vi "SIAM-7xRollingShutter.vi"() -> ()   [LabVIEW 2011]
uses:
  SIAM_command.ctl
panel:
  in  "Wob/µm":dbl=63.28
  in  "Grid µm":dbl=29.0
  out "set Camera Exposure [µs]":dbl=743.175
  in  "PhaseImages":u16=7
  in  "GalvoX-Blanking":dbl
  in  "NoOfImages":u16=35
  out "µmShift":dbl=10.96096971726759 format="%#_8g"
  in  "Camera-Lines":u32=1082
  in  "Turn_ticks":u32=120
  in  "SM_ticks":u32=116
  in  "Trigger_ticks":u32=100
  in  "Mask_tpos":dbl=45853.0
  in  "LineTime-µs":dbl=27.525
  in  "RollingShutter height":u16=27
  in  "galvox/pixel":dbl=7.407
  in  "galvox-Line1080":dbl=-12220.0
  out "SIAMScript":T2(array[cluster])=[{"Delay 10µs"=50, "command"=1612709953, "P0"=0, "P1"=-269103235, "P2"=0, "P3"=0, "P4"=0, "P5-ticket"=0}, {"Delay 10µs"=0, "command"=1611661377, "P0"=0, "P1"=0, "P2"=0, "P3"=0, "P4"=0, "P5-ticket"=0}, {"Delay 10µs"=120, "command"=1612709921, "P0"=0, "P1"=0, "P2"=-2821727, "P3"=0, "P4"=0, "P5-ticket"=0}, {"Delay 10µs"=113, "command"=3506438145, "P0"=1, "P1"=1, "P2"=0, "P3"=0, "P4"=0, "P5-ticket"=0}, {"Delay 10µs"=100, "command"=3506438145, "P0"=1, "P1"=0, "P2"=0, "P3"=0, "P4"=0, "P5-ticket"=0}, {"Delay 10µs"=2856, "command"=1612709921, "P0"=0, "P1"=0, "P2"=0, "P3"=0, "P4"=0, "P5-ticket"=0}, {"Delay 10µs"=50, "command"=1612709953, "P0"=0, "P1"=-269103235, "P2"=0, "P3"=0, "P4"=0, "P5-ticket"=0}, {"Delay 10µs"=0, "command"=1611661377, "P0"=0, "P1"=45250435, "P2"=0, "P3"=0, "P4"=0, "P5-ticket"=0}, {"Delay 10µs"=120, "command"=1612709921, "P0"=0, "P1"=0, "P2"=-2821727, "P3"=0, "P4"=0, "P5-ticket"=0}, {"Delay 10µs"=113, "command"=3506438145, "P0"=1, "P1"=1, "P2"=0, "P3"=0, "P4"=0, "P5-ticket"=0}, {"Delay 10µs"=100, "command"=3506438145, "P0"=1, "P1"=0, "P2"=0, "P3"=0, "P4"=0, "P5-ticket"=0}, {"Delay 10µs"=2856, "command"=1612709921, "P0"=0, "P1"=0, "P2"=0, "P3"=0, "P4"=0, "P5-ticket"=0}, {"Delay 10µs"=50, "command"=1612709953, "P0"=0, "P1"=-269103235, "P2"=0, "P3"=0, "P4"=0, "P5-ticket"=0}, {"Delay 10µs"=0, "command"=1611661377, "P0"=0, "P1"=90500870, "P2"=0, "P3"=0, "P4"=0, "P5-ticket"=0}, {"Delay 10µs"=120, "command"=1612709921, "P0"=0, "P1"=0, "P2"=-2821727, "P3"=0, "P4"=0, "P5-ticket"=0}, {"Delay 10µs"=113, "command"=3506438145, "P0"=1, "P1"=1, "P2"=0, "P3"=0, "P4"=0, "P5-ticket"=0}, {"Delay 10µs"=100, "command"=3506438145, "P0"=1, "P1"=0, "P2"=0, "P3"=0, "P4"=0, "P5-ticket"=0}, {"Delay 10µs"=2856, "command"=1612709921, "P0"=0, "P1"=0, "P2"=0, "P3"=0, "P4"=0, "P5-ticket"=0}, {"Delay 10µs"=50, "command"=1612709953, "P0"=0, "P1"=-269103235, "P2"=0, "P3"=0, "P4"=0, "P5-ticket"=0}, {"Delay 10µs"=0, "command"=1611661377, "P0"=0, "P1"=135751305, "P2"=0, "P3"=0, "P4"=0, "P5-ticket"=0}, {"Delay 10µs"=120, "command"=1612709921, "P0"=0, "P1"=0, "P2"=-2821727, "P3"=0, "P4"=0, "P5-ticket"=0}, {"Delay 10µs"=113, "command"=3506438145, "P0"=1, "P1"=1, "P2"=0, "P3"=0, "P4"=0, "P5-ticket"=0}, {"Delay 10µs"=100, "command"=3506438145, "P0"=1, "P1"=0, "P2"=0, "P3"=0, "P4"=0, "P5-ticket"=0}, {"Delay 10µs"=2856, "command"=1612709921, "P0"=0, "P1"=0, "P2"=0, "P3"=0, "P4"=0, "P5-ticket"=0}, {"Delay 10µs"=50, "command"=1612709953, "P0"=0, "P1"=-269103235, "P2"=0, "P3"=0, "P4"=0, "P5-ticket"=0}, {"Delay 10µs"=0, "command"=1611661377, "P0"=0, "P1"=181001740, "P2"=0, "P3"=0, "P4"=0, "P5-ticket"=0}, {"Delay 10µs"=120, "command"=1612709921, "P0"=0, "P1"=0, "P2"=-2821727, "P3"=0, "P4"=0, "P5-ticket"=0}, {"Delay 10µs"=113, "command"=3506438145, "P0"=1, "P1"=1, "P2"=0, "P3"=0, "P4"=0, "P5-ticket"=0}, {"Delay 10µs"=100, "command"=3506438145, "P0"=1, "P1"=0, "P2"=0, "P3"=0, "P4"=0, "P5-ticket"=0}, {"Delay 10µs"=2856, "command"=1612709921, "P0"=0, "P1"=0, "P2"=0, "P3"=0, "P4"=0, "P5-ticket"=0}, {"Delay 10µs"=50, "command"=1612709953, "P0"=0, "P1"=-269103235, "P2"=0, "P3"=0, "P4"=0, "P5-ticket"=0}, {"Delay 10µs"=0, "command"=1611661377, "P0"=0, "P1"=226252175, "P2"=0, "P3"=0, "P4"=0, "P5-ticket"=0}, {"Delay 10µs"=120, "command"=1612709921, "P0"=0, "P1"=0, "P2"=-2821727, "P3"=0, "P4"=0, "P5-ticket"=0}, {"Delay 10µs"=113, "command"=3506438145, "P0"=1, "P1"=1, "P2"=0, "P3"=0, "P4"=0, "P5-ticket"=0}, {"Delay 10µs"=100, "command"=3506438145, "P0"=1, "P1"=0, "P2"=0, "P3"=0, "P4"=0, "P5-ticket"=0}, {"Delay 10µs"=2856, "command"=1612709921, "P0"=0, "P1"=0, "P2"=0, "P3"=0, "P4"=0, "P5-ticket"=0}, {"Delay 10µs"=50, "command"=1612709953, "P0"=0, "P1"=-269103235, "P2"=0, "P3"=0, "P4"=0, "P5-ticket"=0}, {"Delay 10µs"=0, "command"=1611661377, "P0"=0, "P1"=271502610, "P2"=0, "P3"=0, "P4"=0, "P5-ticket"=0}, {"Delay 10µs"=120, "command"=1612709921, "P0"=0, "P1"=0, "P2"=-2821727, "P3"=0, "P4"=0, "P5-ticket"=0}, {"Delay 10µs"=113, "command"=3506438145, "P0"=1, "P1"=1, "P2"=0, "P3"=0, "P4"=0, "P5-ticket"=0}, {"Delay 10µs"=100, "command"=3506438145, "P0"=1, "P1"=0, "P2"=0, "P3"=0, "P4"=0, "P5-ticket"=0}, {"Delay 10µs"=2856, "command"=1612709921, "P0"=0, "P1"=0, "P2"=0, "P3"=0, "P4"=0, "P5-ticket"=0}, {"Delay 10µs"=50, "command"=1612709953, "P0"=0, "P1"=-269103235, "P2"=0, "P3"=0, "P4"=0, "P5-ticket"=0}, {"Delay 10µs"=0, "command"=1611661377, "P0"=0, "P1"=316753045, "P2"=0, "P3"=0, "P4"=0, "P5-ticket"=0}, {"Delay 10µs"=120, "command"=1612709921, "P0"=0, "P1"=0, "P2"=-2821727, "P3"=0, "P4"=0, "P5-ticket"=0}, {"Delay 10µs"=113, "command"=3506438145, "P0"=1, "P1"=1, "P2"=0, "P3"=0, "P4"=0, "P5-ticket"=0}, {"Delay 10µs"=100, "command"=3506438145, "P0"=1, "P1"=0, "P2"=0, "P3"=0, "P4"=0, "P5-ticket"=0}, {"Delay 10µs"=2856, "command"=1612709921, "P0"=0, "P1"=0, "P2"=0, "P3"=0, "P4"=0, "P5-ticket"=0}, {"Delay 10µs"=50, "command"=1612709953, "P0"=0, "P1"=-269103235, "P2"=0, "P3"=0, "P4"=0, "P5-ticket"=0}, {"Delay 10µs"=0, "command"=1611661377, "P0"=0, "P1"=362003480, "P2"=0, "P3"=0, "P4"=0, "P5-ticket"=0}, {"Delay 10µs"=120, "command"=1612709921, "P0"=0, "P1"=0, "P2"=-2821727, "P3"=0, "P4"=0, "P5-ticket"=0}, {"Delay 10µs"=113, "command"=3506438145, "P0"=1, "P1"=1, "P2"=0, "P3"=0, "P4"=0, "P5-ticket"=0}, {"Delay 10µs"=100, "command"=3506438145, "P0"=1, "P1"=0, "P2"=0, "P3"=0, "P4"=0, "P5-ticket"=0}, {"Delay 10µs"=2856, "command"=1612709921, "P0"=0, "P1"=0, "P2"=0, "P3"=0, "P4"=0, "P5-ticket"=0}, {"Delay 10µs"=50, "command"=1612709953, "P0"=0, "P1"=-269103235, "P2"=0, "P3"=0, "P4"=0, "P5-ticket"=0}, {"Delay 10µs"=0, "command"=1611661377, "P0"=0, "P1"=407253915, "P2"=0, "P3"=0, "P4"=0, "P5-ticket"=0}, {"Delay 10µs"=120, "command"=1612709921, "P0"=0, "P1"=0, "P2"=-2821727, "P3"=0, "P4"=0, "P5-ticket"=0}, {"Delay 10µs"=113, "command"=3506438145, "P0"=1, "P1"=1, "P2"=0, "P3"=0, "P4"=0, "P5-ticket"=0}, {"Delay 10µs"=100, "command"=3506438145, "P0"=1, "P1"=0, "P2"=0, "P3"=0, "P4"=0, "P5-ticket"=0}, {"Delay 10µs"=2856, "command"=1612709921, "P0"=0, "P1"=0, "P2"=0, "P3"=0, "P4"=0, "P5-ticket"=0}, {"Delay 10µs"=50, "command"=1612709953, "P0"=0, "P1"=-269103235, "P2"=0, "P3"=0, "P4"=0, "P5-ticket"=0}, {"Delay 10µs"=0, "command"=1611661377, "P0"=0, "P1"=452504350, "P2"=0, "P3"=0, "P4"=0, "P5-ticket"=0}, {"Delay 10µs"=120, "command"=1612709921, "P0"=0, "P1"=0, "P2"=-2821727, "P3"=0, "P4"=0, "P5-ticket"=0}, {"Delay 10µs"=113, "command"=3506438145, "P0"=1, "P1"=1, "P2"=0, "P3"=0, "P4"=0, "P5-ticket"=0}, {"Delay 10µs"=100, "command"=3506438145, "P0"=1, "P1"=0, "P2"=0, "P3"=0, "P4"=0, "P5-ticket"=0}, {"Delay 10µs"=2856, "command"=1612709921, "P0"=0, "P1"=0, "P2"=0, "P3"=0, "P4"=0, "P5-ticket"=0}, {"Delay 10µs"=50, "command"=1612709953, "P0"=0, "P1"=-269103235, "P2"=0, "P3"=0, "P4"=0, "P5-ticket"=0}, {"Delay 10µs"=0, "command"=1611661377, "P0"=0, "P1"=497754785, "P2"=0, "P3"=0, "P4"=0, "P5-ticket"=0}, {"Delay 10µs"=120, "command"=1612709921, "P0"=0, "P1"=0, "P2"=-2821727, "P3"=0, "P4"=0, "P5-ticket"=0}, {"Delay 10µs"=113, "command"=3506438145, "P0"=1, "P1"=1, "P2"=0, "P3"=0, "P4"=0, "P5-ticket"=0}, {"Delay 10µs"=100, "command"=3506438145, "P0"=1, "P1"=0, "P2"=0, "P3"=0, "P4"=0, "P5-ticket"=0}, {"Delay 10µs"=2856, "command"=1612709921, "P0"=0, "P1"=0, "P2"=0, "P3"=0, "P4"=0, "P5-ticket"=0}, {"Delay 10µs"=50, "command"=1612709953, "P0"=0, "P1"=-269103235, "P2"=0, "P3"=0, "P4"=0, "P5-ticket"=0}, {"Delay 10µs"=0, "command"=1611661377, "P0"=0, "P1"=543005220, "P2"=0, "P3"=0, "P4"=0, "P5-ticket"=0}, {"Delay 10µs"=120, "command"=1612709921, "P0"=0, "P1"=0, "P2"=-2821727, "P3"=0, "P4"=0, "P5-ticket"=0}, {"Delay 10µs"=113, "command"=3506438145, "P0"=1, "P1"=1, "P2"=0, "P3"=0, "P4"=0, "P5-ticket"=0}, {"Delay 10µs"=100, "command"=3506438145, "P0"=1, "P1"=0, "P2"=0, "P3"=0, "P4"=0, "P5-ticket"=0}, {"Delay 10µs"=2856, "command"=1612709921, "P0"=0, "P1"=0, "P2"=0, "P3"=0, "P4"=0, "P5-ticket"=0}, {"Delay 10µs"=50, "command"=1612709953, "P0"=0, "P1"=-269103235, "P2"=0, "P3"=0, "P4"=0, "P5-ticket"=0}, {"Delay 10µs"=0, "command"=1611661377, "P0"=0, "P1"=588255655, "P2"=0, "P3"=0, "P4"=0, "P5-ticket"=0}, {"Delay 10µs"=120, "command"=1612709921, "P0"=0, "P1"=0, "P2"=-2821727, "P3"=0, "P4"=0, "P5-ticket"=0}, {"Delay 10µs"=113, "command"=3506438145, "P0"=1, "P1"=1, "P2"=0, "P3"=0, "P4"=0, "P5-ticket"=0}, {"Delay 10µs"=100, "command"=3506438145, "P0"=1, "P1"=0, "P2"=0, "P3"=0, "P4"=0, "P5-ticket"=0}, {"Delay 10µs"=2856, "command"=1612709921, "P0"=0, "P1"=0, "P2"=0, "P3"=0, "P4"=0, "P5-ticket"=0}, {"Delay 10µs"=50, "command"=1612709953, "P0"=0, "P1"=-269103235, "P2"=0, "P3"=0, "P4"=0, "P5-ticket"=0}, {"Delay 10µs"=0, "command"=1611661377, "P0"=0, "P1"=633506090, "P2"=0, "P3"=0, "P4"=0, "P5-ticket"=0}, {"Delay 10µs"=120, "command"=1612709921, "P0"=0, "P1"=0, "P2"=-2821727, "P3"=0, "P4"=0, "P5-ticket"=0}, {"Delay 10µs"=113, "command"=3506438145, "P0"=1, "P1"=1, "P2"=0, "P3"=0, "P4"=0, "P5-ticket"=0}, {"Delay 10µs"=100, "command"=3506438145, "P0"=1, "P1"=0, "P2"=0, "P3"=0, "P4"=0, "P5-ticket"=0}, {"Delay 10µs"=2856, "command"=1612709921, "P0"=0, "P1"=0, "P2"=0, "P3"=0, "P4"=0, "P5-ticket"=0}, {"Delay 10µs"=50, "command"=1612709953, "P0"=0, "P1"=-269103235, "P2"=0, "P3"=0, "P4"=0, "P5-ticket"=0}, {"Delay 10µs"=0, "command"=1611661377, "P0"=0, "P1"=678756525, "P2"=0, "P3"=0, "P4"=0, "P5-ticket"=0}, {"Delay 10µs"=120, "command"=1612709921, "P0"=0, "P1"=0, "P2"=-2821727, "P3"=0, "P4"=0, "P5-ticket"=0}, {"Delay 10µs"=113, "command"=3506438145, "P0"=1, "P1"=1, "P2"=0, "P3"=0, "P4"=0, "P5-ticket"=0}, {"Delay 10µs"=100, "command"=3506438145, "P0"=1, "P1"=0, "P2"=0, "P3"=0, "P4"=0, "P5-ticket"=0}, {"Delay 10µs"=2856, "command"=1612709921, "P0"=0, "P1"=0, "P2"=0, "P3"=0, "P4"=0, "P5-ticket"=0}, {"Delay 10µs"=50, "command"=1612709953, "P0"=0, "P1"=-269103235, "P2"=0, "P3"=0, "P4"=0, "P5-ticket"=0}, {"Delay 10µs"=0, "command"=1611661377, "P0"=0, "P1"=724006960, "P2"=0, "P3"=0, "P4"=0, "P5-ticket"=0}, {"Delay 10µs"=120, "command"=1612709921, "P0"=0, "P1"=0, "P2"=-2821727, "P3"=0, "P4"=0, "P5-ticket"=0}, {"Delay 10µs"=113, "command"=3506438145, "P0"=1, "P1"=1, "P2"=0, "P3"=0, "P4"=0, "P5-ticket"=0}, {"Delay 10µs"=100, "command"=3506438145, "P0"=1, "P1"=0, "P2"=0, "P3"=0, "P4"=0, "P5-ticket"=0}, {"Delay 10µs"=2856, "command"=1612709921, "P0"=0, "P1"=0, "P2"=0, "P3"=0, "P4"=0, "P5-ticket"=0}, {"Delay 10µs"=50, "command"=1612709953, "P0"=0, "P1"=-269103235, "P2"=0, "P3"=0, "P4"=0, "P5-ticket"=0}, {"Delay 10µs"=0, "command"=1611661377, "P0"=0, "P1"=769257395, "P2"=0, "P3"=0, "P4"=0, "P5-ticket"=0}, {"Delay 10µs"=120, "command"=1612709921, "P0"=0, "P1"=0, "P2"=-2821727, "P3"=0, "P4"=0, "P5-ticket"=0}, {"Delay 10µs"=113, "command"=3506438145, "P0"=1, "P1"=1, "P2"=0, "P3"=0, "P4"=0, "P5-ticket"=0}, {"Delay 10µs"=100, "command"=3506438145, "P0"=1, "P1"=0, "P2"=0, "P3"=0, "P4"=0, "P5-ticket"=0}, {"Delay 10µs"=2856, "command"=1612709921, "P0"=0, "P1"=0, "P2"=0, "P3"=0, "P4"=0, "P5-ticket"=0}, {"Delay 10µs"=50, "command"=1612709953, "P0"=0, "P1"=-269103235, "P2"=0, "P3"=0, "P4"=0, "P5-ticket"=0}, {"Delay 10µs"=0, "command"=1611661377, "P0"=0, "P1"=814507830, "P2"=0, "P3"=0, "P4"=0, "P5-ticket"=0}, {"Delay 10µs"=120, "command"=1612709921, "P0"=0, "P1"=0, "P2"=-2821727, "P3"=0, "P4"=0, "P5-ticket"=0}, {"Delay 10µs"=113, "command"=3506438145, "P0"=1, "P1"=1, "P2"=0, "P3"=0, "P4"=0, "P5-ticket"=0}, {"Delay 10µs"=100, "command"=3506438145, "P0"=1, "P1"=0, "P2"=0, "P3"=0, "P4"=0, "P5-ticket"=0}, {"Delay 10µs"=2856, "command"=1612709921, "P0"=0, "P1"=0, "P2"=0, "P3"=0, "P4"=0, "P5-ticket"=0}, {"Delay 10µs"=50, "command"=1612709953, "P0"=0, "P1"=-269103235, "P2"=0, "P3"=0, "P4"=0, "P5-ticket"=0}, {"Delay 10µs"=0, "command"=1611661377, "P0"=0, "P1"=859758265, "P2"=0, "P3"=0, "P4"=0, "P5-ticket"=0}, {"Delay 10µs"=120, "command"=1612709921, "P0"=0, "P1"=0, "P2"=-2821727, "P3"=0, "P4"=0, "P5-ticket"=0}, {"Delay 10µs"=113, "command"=3506438145, "P0"=1, "P1"=1, "P2"=0, "P3"=0, "P4"=0, "P5-ticket"=0}, {"Delay 10µs"=100, "command"=3506438145, "P0"=1, "P1"=0, "P2"=0, "P3"=0, "P4"=0, "P5-ticket"=0}, {"Delay 10µs"=2856, "command"=1612709921, "P0"=0, "P1"=0, "P2"=0, "P3"=0, "P4"=0, "P5-ticket"=0}, {"Delay 10µs"=50, "command"=1612709953, "P0"=0, "P1"=-269103235, "P2"=0, "P3"=0, "P4"=0, "P5-ticket"=0}, {"Delay 10µs"=0, "command"=1611661377, "P0"=0, "P1"=905008700, "P2"=0, "P3"=0, "P4"=0, "P5-ticket"=0}, {"Delay 10µs"=120, "command"=1612709921, "P0"=0, "P1"=0, "P2"=-2821727, "P3"=0, "P4"=0, "P5-ticket"=0}, {"Delay 10µs"=113, "command"=3506438145, "P0"=1, "P1"=1, "P2"=0, "P3"=0, "P4"=0, "P5-ticket"=0}, {"Delay 10µs"=100, "command"=3506438145, "P0"=1, "P1"=0, "P2"=0, "P3"=0, "P4"=0, "P5-ticket"=0}, {"Delay 10µs"=2856, "command"=1612709921, "P0"=0, "P1"=0, "P2"=0, "P3"=0, "P4"=0, "P5-ticket"=0}, {"Delay 10µs"=50, "command"=1612709953, "P0"=0, "P1"=-269103235, "P2"=0, "P3"=0, "P4"=0, "P5-ticket"=0}, {"Delay 10µs"=0, "command"=1611661377, "P0"=0, "P1"=950259135, "P2"=0, "P3"=0, "P4"=0, "P5-ticket"=0}, {"Delay 10µs"=120, "command"=1612709921, "P0"=0, "P1"=0, "P2"=-2821727, "P3"=0, "P4"=0, "P5-ticket"=0}, {"Delay 10µs"=113, "command"=3506438145, "P0"=1, "P1"=1, "P2"=0, "P3"=0, "P4"=0, "P5-ticket"=0}, {"Delay 10µs"=100, "command"=3506438145, "P0"=1, "P1"=0, "P2"=0, "P3"=0, "P4"=0, "P5-ticket"=0}, {"Delay 10µs"=2856, "command"=1612709921, "P0"=0, "P1"=0, "P2"=0, "P3"=0, "P4"=0, "P5-ticket"=0}, {"Delay 10µs"=50, "command"=1612709953, "P0"=0, "P1"=-269103235, "P2"=0, "P3"=0, "P4"=0, "P5-ticket"=0}, {"Delay 10µs"=0, "command"=1611661377, "P0"=0, "P1"=995509570, "P2"=0, "P3"=0, "P4"=0, "P5-ticket"=0}, {"Delay 10µs"=120, "command"=1612709921, "P0"=0, "P1"=0, "P2"=-2821727, "P3"=0, "P4"=0, "P5-ticket"=0}, {"Delay 10µs"=113, "command"=3506438145, "P0"=1, "P1"=1, "P2"=0, "P3"=0, "P4"=0, "P5-ticket"=0}, {"Delay 10µs"=100, "command"=3506438145, "P0"=1, "P1"=0, "P2"=0, "P3"=0, "P4"=0, "P5-ticket"=0}, {"Delay 10µs"=2856, "command"=1612709921, "P0"=0, "P1"=0, "P2"=0, "P3"=0, "P4"=0, "P5-ticket"=0}, {"Delay 10µs"=50, "command"=1612709953, "P0"=0, "P1"=-269103235, "P2"=0, "P3"=0, "P4"=0, "P5-ticket"=0}, {"Delay 10µs"=0, "command"=1611661377, "P0"=0, "P1"=1040760005, "P2"=0, "P3"=0, "P4"=0, "P5-ticket"=0}, {"Delay 10µs"=120, "command"=1612709921, "P0"=0, "P1"=0, "P2"=-2821727, "P3"=0, "P4"=0, "P5-ticket"=0}, {"Delay 10µs"=113, "command"=3506438145, "P0"=1, "P1"=1, "P2"=0, "P3"=0, "P4"=0, "P5-ticket"=0}, {"Delay 10µs"=100, "command"=3506438145, "P0"=1, "P1"=0, "P2"=0, "P3"=0, "P4"=0, "P5-ticket"=0}, {"Delay 10µs"=2856, "command"=1612709921, "P0"=0, "P1"=0, "P2"=0, "P3"=0, "P4"=0, "P5-ticket"=0}, {"Delay 10µs"=50, "command"=1612709953, "P0"=0, "P1"=-269103235, "P2"=0, "P3"=0, "P4"=0, "P5-ticket"=0}, {"Delay 10µs"=0, "command"=1611661377, "P0"=0, "P1"=1086010440, "P2"=0, "P3"=0, "P4"=0, "P5-ticket"=0}, {"Delay 10µs"=120, "command"=1612709921, "P0"=0, "P1"=0, "P2"=-2821727, "P3"=0, "P4"=0, "P5-ticket"=0}, {"Delay 10µs"=113, "command"=3506438145, "P0"=1, "P1"=1, "P2"=0, "P3"=0, "P4"=0, "P5-ticket"=0}, {"Delay 10µs"=100, "command"=3506438145, "P0"=1, "P1"=0, "P2"=0, "P3"=0, "P4"=0, "P5-ticket"=0}, {"Delay 10µs"=2856, "command"=1612709921, "P0"=0, "P1"=0, "P2"=0, "P3"=0, "P4"=0, "P5-ticket"=0}, {"Delay 10µs"=50, "command"=1612709953, "P0"=0, "P1"=0, "P2"=0, "P3"=0, "P4"=0, "P5-ticket"=0}, {"Delay 10µs"=10, "command"=4027518991, "P0"=0, "P1"=0, "P2"=0, "P3"=0, "P4"=0, "P5-ticket"=12345}] {"command" format="%x" items=["read_x-Motor_status_ticket"=17305600, "init_x-Motor"=17760263, "read_x-Motor_absolute_ticket"=16781312, "move_x-Motor_absolute"=16777217, "move_x-Motor_relative"=16842753, "read_y-Motor_status_ticket"=18354176, "init_y-Motor"=18808839, "read_y-Motor_absolute_ticket"=17829888, "move_y-Motor_absolute"=17825793, "move_y-Motor_relative"=17891329, "read_z-Motor_status_ticket"=19402752, "init_z-Motor"=19857415, "stop_z-Motor"=19857423, "start_z-Motor"=19857422, "read_z-Motor_absolute_ticket"=18878464, "move_z-Motor_absolute"=18874369, "move_z-Motor_relative"=18939905, "end_no_ticket"=4027514895, "end_ticket"=4027518991, "IO-read_bank0"=3489665024, "IO-write_bank0"=3489660929, "IO-read_bank1"=3506442240, "IO-write_bank1"=3506438145, "Analog-write_DA0-0"=2684354561, "Analog-write_DA0-1"=2685403137, "Analog-write_DA0-2"=2686451713, "Analog-write_DA0-3"=2687500289, "Analog-write_DA0-4"=2688548865, "Analog-write_DA0-5"=2689597441, "Analog-write_DA0-6"=2690646017, "Analog-write_DA0-7"=2691694593, "Analog-write_DA1-0"=2701131777, "Analog-write_DA1-1"=2702180353, "Analog-write_DA1-2"=2703228929, "Analog-write_DA1-3"=2704277505, "Analog-write_DA1-4"=2705326081, "Analog-write_DA1-5"=2706374657, "Analog-write_DA1-6"=2707423233, "Analog-write_DA1-7"=2708471809, "Analog-read_AD0-0"=2818576384, "Analog-read-store_AD0-0"=2818572290, "IO-delay_bank0"=3489923073, "IO-delay_bank0_fromVar"=3489923075, "read_cam_clock"=3289124864, "store_cam_clock"=3289120770, "read_cam_phase"=3289190400, "set_cam_deadtime"=3288989697, "set_cam_10uscycles"=3289055233, "set_cam_10uscycles_fromVariable"=3289055235, "calc_cam"=3289317386, "store_cam_Var"=3289251842, "math_addToVariable"=4060086278, "readVar"=4060090368, "writeVar"=4060086273, "copyVar"=4060086276, "decrement_branchRel_if_equal"=4043374945, "decrement_branchRel_if_greaterequal"=4043375201, "decrement_branchRel_if_greaterequal_withTicket"=4043379297, "decrement_branchRel_if_smaller"=4043375457, "increment_branchRel_if_smaller"=4043375473, "set_x-Galvo"=1612710129, "set_y-Galvo"=1613758705, "set_z-Fokus"=1614807281, "set_x-Galvo_position-only"=1612709953, "set_y-Galvo_position-only"=1613758529, "set_z-Fokus_position-only"=1614807105, "set_x-Galvo_position-only_ticket"=1612714049, "set_y-Galvo_position-only_ticket"=1613762625, "set_z-Fokus_position-only_ticket"=1614811201, "set_x-Galvo_speed-only"=1612709921, "set_y-Galvo_speed-only"=1613758497, "set_z-Fokus_speed-only"=1614807073, "read_x-Galvo_ticket"=1612714048, "read_y-Galvo_ticket"=1613762624, "read_z-Focus_ticket"=1614811200, "x-Galvo_pos_fromVar"=1612709955, "y-Galvo_pos_fromVar"=1613758531, "z-Focus_pos_fromVar"=1614807107]}
  # "jetzt x-wob orthogonal"
  # "29er/7=45250435"
  # "22/25,5/29"
  # "12,75+-0,02"
  # "12,75: 25,5\n14,4956: 29er"
  # "29 full wobbel=4833,267908cnt\n/sqrt(7) =1826,803557\n/29=62,993226 wob/µm"
  # "Zum einstellnen der 19.1°\ngemessen +0,0068°/step, 0bei 291,6°\ntheorie +0,00703°/step"
  # "tilcal 1\nspeed 50\nidmax"
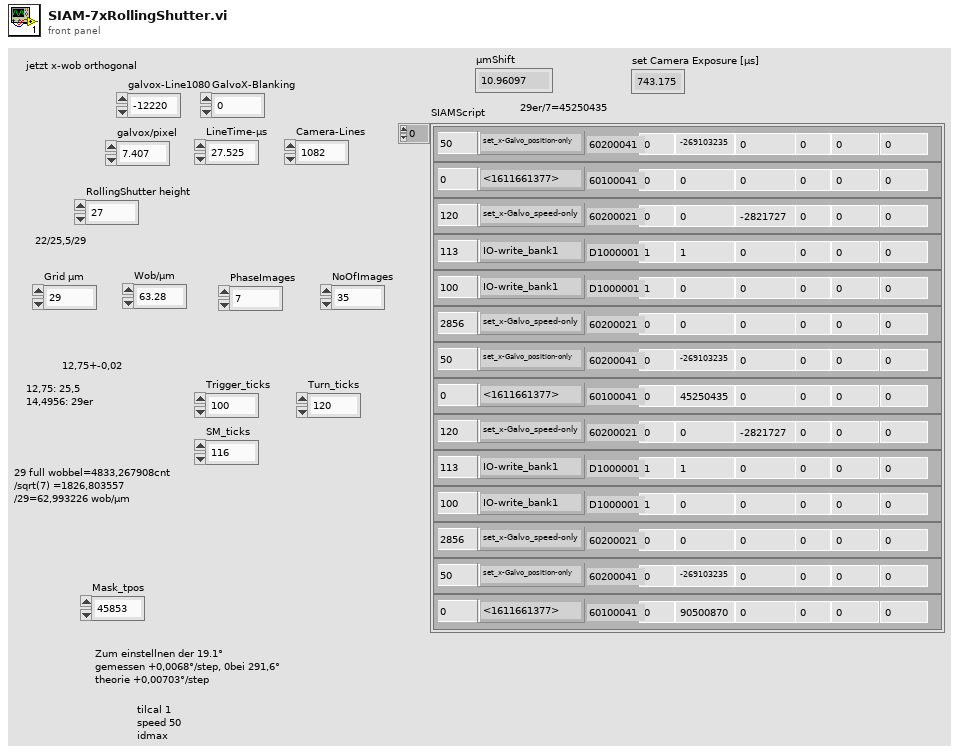
[diagram p1: front panel]
types:
  T1 = typedef "SIAM_command.ctl" = u32
  T2 = cluster{"Delay 10µs":u32, "command":T1, "P0":i32, "P1":i32, "P2":i32, "P3":i32, "P4":i32, "P5-ticket":i32}[]
  T3 = enum8{"Ch0", "Ch1", "x-Galvo", "y-Galvo", "z-Focus"}
  T4 = cluster{"Delay 10µs":u32, "command":T1, "P0":i32, "P1":i32, "P2":i32, "P3":i32, "P4":i32, "P5-ticket":i32}
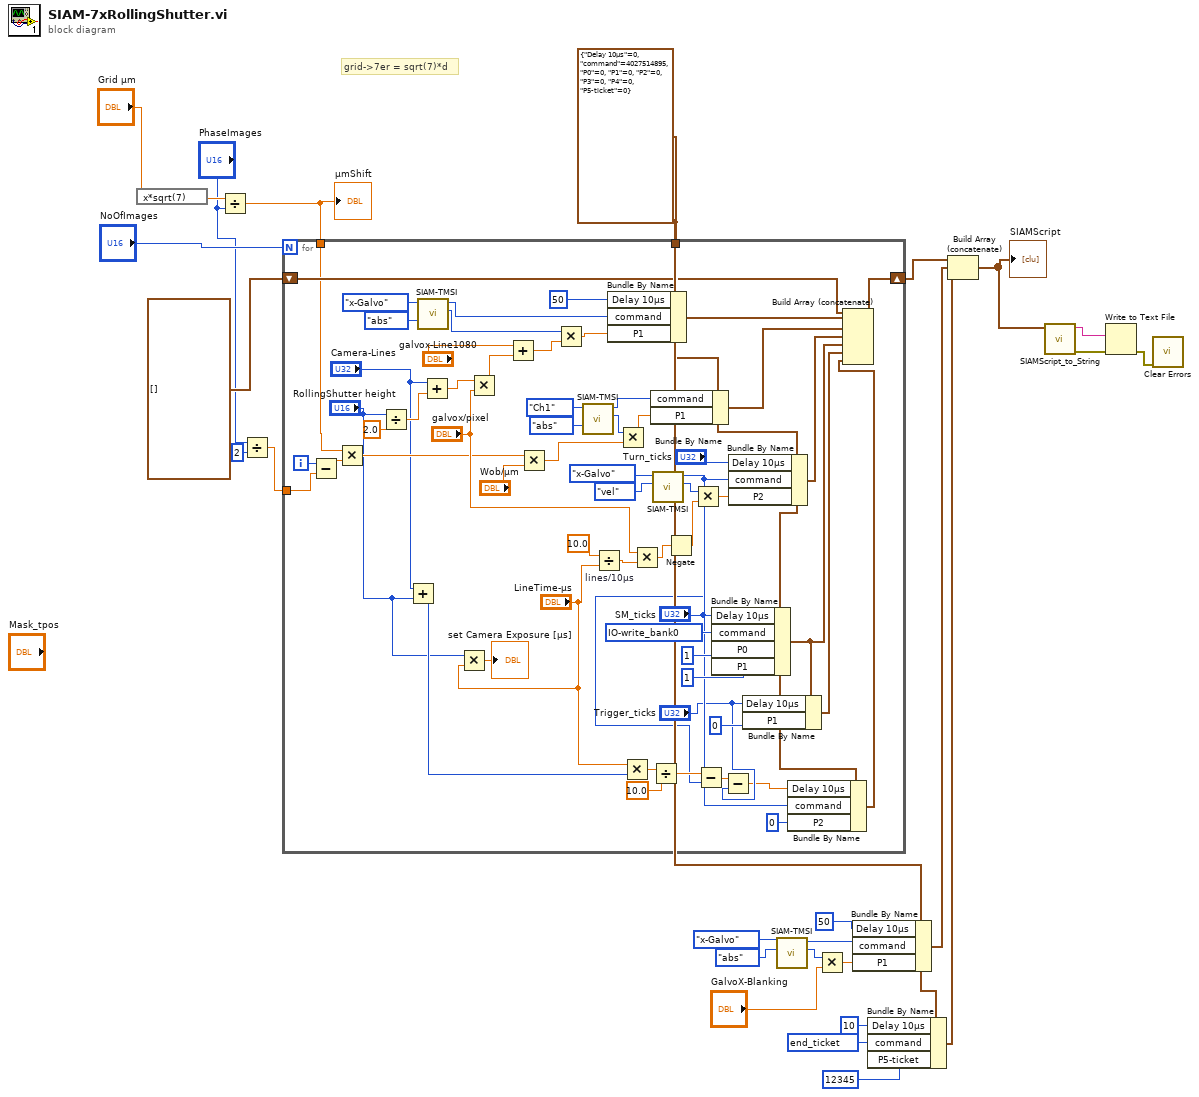
[diagram p0: block diagram]
diagram:
  w13 = T1 4027518991 items=["read_x-Motor_status_ticket"=17305600, "init_x-Motor"=17760263, "read_x-Motor_absolute_ticket"=16781312, "move_x-Motor_absolute"=16777217, "move_x-Motor_relative"=16842753, "read_y-Motor_status_ticket"=18354176, "init_y-Motor"=18808839, "read_y-Motor_absolute_ticket"=17829888, "move_y-Motor_absolute"=17825793, "move_y-Motor_relative"=17891329, "read_z-Motor_status_ticket"=19402752, "init_z-Motor"=19857415, "stop_z-Motor"=19857423, "start_z-Motor"=19857422, "read_z-Motor_absolute_ticket"=18878464, "move_z-Motor_absolute"=18874369, "move_z-Motor_relative"=18939905, "end_no_ticket"=4027514895, "end_ticket"=4027518991, "IO-read_bank0"=3489665024, "IO-write_bank0"=3489660929, "IO-read_bank1"=3506442240, "IO-write_bank1"=3506438145, "IO-delay_bank0"=3489923073, "IO-delay_bank0_fromVar"=3489923075, "read_cam_clock"=3289124864, "store_cam_clock"=3289120770, "read_cam_phase"=3289190400, "set_cam_deadtime"=3288989697, "set_cam_10uscycles"=3289055233, "set_cam_10uscycles_fromVariable"=3289055235, "calc_cam"=3289317386, "store_cam_Var"=3289251842, "math_addToVariable"=4060086278, "readVar"=4060090368, "writeVar"=4060086273, "copyVar"=4060086276, "decrement_branchRel_if_equal"=4043374945, "decrement_branchRel_if_greaterequal"=4043375201, "decrement_branchRel_if_greaterequal_withTicket"=4043379297, "decrement_branchRel_if_smaller"=4043375457, "increment_branchRel_if_smaller"=4043375473, "set_x-Galvo"=1612710129, "set_y-Galvo"=1613758705, "set_z-Fokus"=1614807281, "set_x-Galvo_position-only"=1612709953, "set_y-Galvo_position-only"=1613758529, "set_z-Fokus_position-only"=1614807105, "set_x-Galvo_position-only_ticket"=1612714049, "set_y-Galvo_position-only_ticket"=1613762625, "set_z-Fokus_position-only_ticket"=1614811201, "read_x-Galvo_ticket"=1612714048, "read_y-Galvo_ticket"=1613762624, "read_z-Focus_ticket"=1614811200, "x-Galvo_pos_fromVar"=1612709955, "y-Galvo_pos_fromVar"=1613758531, "z-Focus_pos_fromVar"=1614807107] ("command")
  w14 = T4 {"Delay 10µs"=0, "command"=4027514895, "P0"=0, "P1"=0, "P2"=0, "P3"=0, "P4"=0, "P5-ticket"=0} ("Cluster")
  # "grid->7er = sqrt(7)*d"
  n1 = expression code="x*sqrt(7)"("Grid µm") -> (w4:dbl)
  n2 = Divide(x=w4, y="PhaseImages") -> (x/y=w23:dbl)
  "µmShift" <- w23
  n3 = Divide(x="PhaseImages", y=u16 2) -> (x/y=w1:dbl)
  n4 = for {
    N: "NoOfImages" -> [_]
    tunnel: w23 -> [w39]
    tunnel: w14 -> [w54]
    shift-right: [w43] -> w25
    shift-left: T2 [] -> [w42]
    tunnel: w1 -> [w27]
    i -> [w40]
    w60 = T1 3489660929 items=["read_x-Motor_status_ticket"=17305600, "init_x-Motor"=17760263, "read_x-Motor_absolute_ticket"=16781312, "move_x-Motor_absolute"=16777217, "move_x-Motor_relative"=16842753, "read_y-Motor_status_ticket"=18354176, "init_y-Motor"=18808839, "read_y-Motor_absolute_ticket"=17829888, "move_y-Motor_absolute"=17825793, "move_y-Motor_relative"=17891329, "read_z-Motor_status_ticket"=19402752, "init_z-Motor"=19857415, "stop_z-Motor"=19857423, "start_z-Motor"=19857422, "read_z-Motor_absolute_ticket"=18878464, "move_z-Motor_absolute"=18874369, "move_z-Motor_relative"=18939905, "end_no_ticket"=4027514895, "end_ticket"=4027518991, "IO-read_bank0"=3489665024, "IO-write_bank0"=3489660929, "IO-read_bank1"=3506442240, "IO-write_bank1"=3506438145, "IO-delay_bank0"=3489923073, "IO-delay_bank0_fromVar"=3489923075, "read_cam_clock"=3289124864, "store_cam_clock"=3289120770, "read_cam_phase"=3289190400, "set_cam_deadtime"=3288989697, "set_cam_10uscycles"=3289055233, "set_cam_10uscycles_fromVariable"=3289055235, "calc_cam"=3289317386, "store_cam_Var"=3289251842, "math_addToVariable"=4060086278, "readVar"=4060090368, "writeVar"=4060086273, "copyVar"=4060086276, "decrement_branchRel_if_equal"=4043374945, "decrement_branchRel_if_greaterequal"=4043375201, "decrement_branchRel_if_greaterequal_withTicket"=4043379297, "decrement_branchRel_if_smaller"=4043375457, "increment_branchRel_if_smaller"=4043375473, "set_x-Galvo"=1612710129, "set_y-Galvo"=1613758705, "set_z-Fokus"=1614807281, "set_x-Galvo_position-only"=1612709953, "set_y-Galvo_position-only"=1613758529, "set_z-Fokus_position-only"=1614807105, "set_x-Galvo_position-only_ticket"=1612714049, "set_y-Galvo_position-only_ticket"=1613762625, "set_z-Fokus_position-only_ticket"=1614811201, "read_x-Galvo_ticket"=1612714048, "read_y-Galvo_ticket"=1613762624, "read_z-Focus_ticket"=1614811200, "x-Galvo_pos_fromVar"=1612709955, "y-Galvo_pos_fromVar"=1613758531, "z-Focus_pos_fromVar"=1614807107] ("command")
    n5 = Subtract(x=w40, y=w27) -> (x-y=w28:dbl)
    n6 = Multiply(x=w39, y=w28) -> (x*y=w38:dbl)
    n7 = Divide(x="RollingShutter height", y=2.0) -> (x/y=w83:dbl)
    n8 = Add(x="Camera-Lines", y="RollingShutter height") -> (x+y=w35:u32)
    n9 = call "SIAM-TMSI.vi"("Type"=enum8{"acc", "vel", "abs", "offset"}."abs", "Motor"=T3."x-Galvo") -> ("Resolution-Factor"=w79:i32, "command"=w85:T1)  [unwired: 6 in, 2 out]
    n10 = Add(x="Camera-Lines", y=w83) -> (x+y=w30:dbl)
    n11 = Multiply(x="RollingShutter height", y="LineTime-µs") -> (x*y=→"set Camera Exposure [µs]":dbl)
    n12 = Multiply(x=w30, y="galvox/pixel") -> (x*y=w82:dbl)
    n13 = Add(x="galvox-Line1080", y=w82) -> (x+y=w80:dbl)
    n14 = Multiply(x=w38, y="Wob/µm") -> (x*y=w71:dbl)
    n15 = Multiply(x=w79, y=w80) -> (x*y=w78:dbl)
    n16 = call "SIAM-TMSI.vi"("Type"=enum8{"acc", "vel", "abs", "offset"}."abs", "Motor"=T3."Ch1") -> ("Resolution-Factor"=w72:i32, "command"=w73:T1)  [unwired: 6 in, 2 out]
    n17 = Divide "lines/10µs"(x=10.0 ("y"), y="LineTime-µs") -> (x/y=w63:dbl)
    n18 = Bundle By Name(cluster=w54, "Delay 10µs"=u32 50, "command"=w85, "P1"=w78) -> (w77:T4)
    n19 = Multiply(x=w72, y=w71) -> (x*y=w70:dbl)
    n20 = Multiply(x="LineTime-µs", y=w35) -> (x*y=w51:dbl)
    n21 = Multiply(x="galvox/pixel", y=w63) -> (x*y=w61:dbl)
    n22 = Bundle By Name(cluster=w54, "command"=w73, "P1"=w70) -> (w76:T4)
    n23 = Divide(x=w51, y=10.0) -> (x/y=w49:dbl)
    n24 = call "SIAM-TMSI.vi"("Type"=enum8{"acc", "vel", "abs", "offset"}."vel", "Motor"=T3."x-Galvo") -> ("Resolution-Factor"=w65:i32, "command"=w52:T1)  [unwired: 6 in, 2 out]
    n25 = Negate(x=w61) -> (-x=w41:dbl)
    n26 = Multiply(x=w65, y=w41) -> (x*y=w66:dbl)
    n27 = Subtract(x=w49, y="SM_ticks") -> (x-y=w47:dbl)
    n28 = Bundle By Name(cluster=w54, "Delay 10µs"="SM_ticks", "command"=w60, "P0"=1, "P1"=1) -> (w57:T4)
    n29 = Subtract(x=w47, y="Trigger_ticks") -> (x-y=w45:dbl)
    n30 = Bundle By Name(cluster=w54, "Delay 10µs"="Turn_ticks", "command"=w52, "P2"=w66) -> (w67:T4)
    n31 = Bundle By Name(cluster=w57, "Delay 10µs"="Trigger_ticks", "P1"=0) -> (w55:T4)
    n32 = Bundle By Name(cluster=w54, "Delay 10µs"=w45, "command"=w52, "P2"=0) -> (w44:T4)
    n33 = Build Array (concatenate)(w42, w77, w76, w67, w57, w55, w44) -> (w43:T2)
  }
  n34 = call "SIAM-TMSI.vi"("Type"=enum8{"acc", "vel", "abs", "offset"}."abs", "Motor"=T3."x-Galvo") -> ("Resolution-Factor"=w19:i32, "command"=w18:T1)  [unwired: 6 in, 2 out]
  n35 = Multiply(x=w19, y="GalvoX-Blanking") -> (x*y=w20:dbl)
  n36 = Bundle By Name(cluster=w14, "Delay 10µs"=u32 50, "command"=w18, "P1"=w20) -> (w15:T4)
  n37 = Bundle By Name(cluster=w14, "Delay 10µs"=u32 10, "command"=w13, "P5-ticket"=12345) -> (w11:T4)
  n38 = Build Array (concatenate)(w25, w15, w11) -> (w9:T2)
  "SIAMScript" <- w9
  n39 = call "SIAMScript_to_String.vi"("Script"=w9) -> ("error out"=w7:errorcluster, "String"=w8:string)  [unwired: 9 in]
  n40 = Write to Text File(text=w8, error in=w7) -> (error out=w6:errorcluster)  [unwired: 2 in, 2 out]
  n41 = call <vilib>:"Clear Errors.vi"("error in (no error)"=w6) -> ()  [unwired: 6 in, 1 out]
